vi "CMD_Processor.vi"(8 "error in (no error)":errorcluster, 10 "objects in":T1, 11 "value":variant) -> (0 "error out":errorcluster, 3 "objects out":T1)   [LabVIEW 2025]
uses:
  Classes/Processor/Processor.lvclass
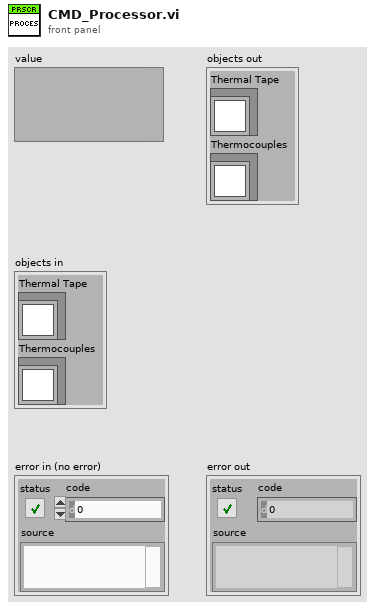
[diagram p1: front panel]
types:
  T1 = cluster{"Thermal Tape":refnum<class "Processor.lvclass">, "Thermocouples":refnum<class "Processor.lvclass">}
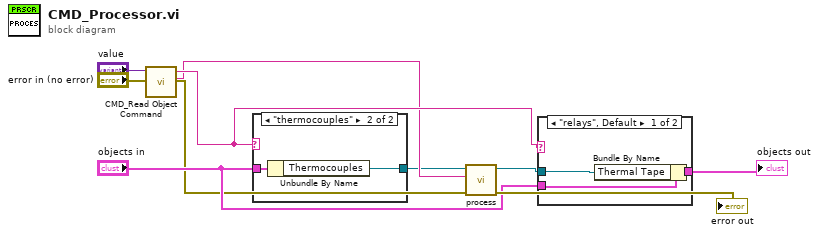
[diagram p0: block diagram]
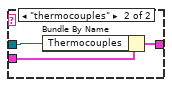
[diagram p2: hidden frame]
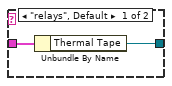
[diagram p3: hidden frame]
diagram:
  n1 = call "CMD_Read Object Command.vi"("value"="value") -> ("Command"=w4:string, "Object"=w5:string)  [unwired: 9 in]
  n2 = case shown="\"thermocouples\"" w5 {
    tunnel: "objects in" -> [w11 w13]
    tunnel: [w10 w12] -> w2
    frame "relays", Default {
      n3 = Unbundle By Name(w11) -> ("Thermal Tape"=w10:refnum<class "Processor.lvclass">)
    }
    frame "thermocouples" {
      n4 = Unbundle By Name(w13) -> ("Thermocouples"=w12:refnum<class "Processor.lvclass">)
    }
  }
  n5 = call-dynamic "process.vi"("error in (no error)"="error in (no error)", "Process"=w4, "Processor in"=w2) -> ("error out"=→"error out":errorcluster, "Processor out"=w7:refnum<class "Processor.lvclass">)  [unwired: 7 in]
  n6 = case shown="\"relays\", Default" w5 {
    tunnel: w7 -> [w14 w17]
    tunnel: [w16 w19] -> w8
    tunnel: "objects in" -> [w15 w18]
    frame "relays", Default {
      n7 = Bundle By Name(cluster=w15, "Thermal Tape"=w14) -> (w16:T1)
    }
    frame "thermocouples" {
      n8 = Bundle By Name(cluster=w18, "Thermocouples"=w17) -> (w19:T1)
    }
  }
  "objects out" <- w8
